vi "VH4TM.vi"(10 "M":dbl, 11 "T":dbl[unit]) -> (1 "S":dbl[unit], 2 "V":dbl[unit], 3 "H":dbl[unit])   [LabVIEW 2011]
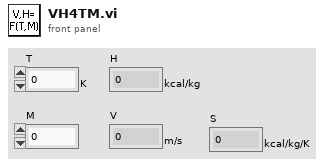
[diagram p1: front panel]
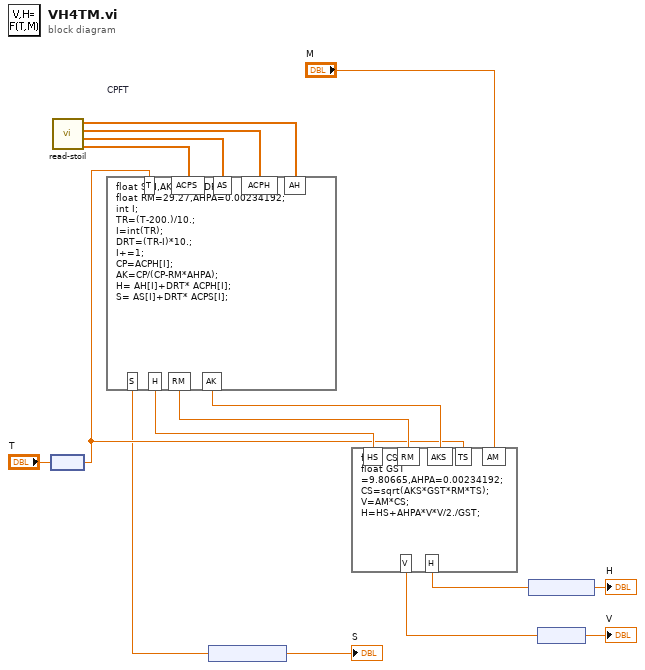
[diagram p0: block diagram]
diagram:
  n1 = node("T") -> (w5:dbl)
  n2 = call "read-stoil.vi"() -> ("ACPS"=w9:dbl[], "AS"=w8:dbl[], "ACPH"=w7:dbl[], "AH"=w6:dbl[])  [unwired: 8 in]
  n3 = formula code="float S,H,AK,CP,TR,DRT;\nfloat RM=29.27,AHPA=0.00234192;\nint I;\nTR=(T-200.)/10.;\nI=int(TR); \nDRT=(TR-I)*10.;\nI+=1;\nCP=ACPH[I];\nAK=CP/(CP-RM*AHPA);\nH= AH[I]+DRT* ACPH[I];\nS= AS[I]+DRT* ACPS[I];" "CPFT"("T"=w5, "AH"=w6, "ACPH"=w7, "AS"=w8, "ACPS"=w9) -> ("S"=w2:dbl, "AK"=w10:dbl, "RM"=w11:dbl, "H"=w14:dbl)
  n4 = node(w2) -> (→"S":dbl[unit])
  n5 = formula code="float CS,V,H;\nfloat GST =9.80665,AHPA=0.00234192;\nCS=sqrt(AKS*GST*RM*TS);\nV=AM*CS;\nH=HS+AHPA*V*V/2./GST;"("AKS"=w10, "RM"=w11, "TS"=w5, "AM"="M", "HS"=w14) -> ("V"=w16:dbl, "H"=w15:dbl)
  n6 = node(w15) -> (→"H":dbl[unit])
  n7 = node(w16) -> (→"V":dbl[unit])
